vi "commander5.vi"() -> ()   [LabVIEW 2015]
uses:
  G_SEN.vi
  G_NAV.vi
  G_DATA.vi
  G_LCM.vi
  G_VEH.vi
  G_PATH.vi
panel:
  in  "shifthold":dbl=0.0025
  out "String":string="콜 서비스 대기 중"
  out "EURECAR_VISION":T1
  out "count":i32
  out "P2V Sign":picture[](array[picture])=[bytes[7530], bytes[7530], bytes[7530], bytes[7530]]
  out "Array 2":picture[](array[picture])
  out "sign 2":picture[](array[picture])
  out "sign":picture[](array[picture])
  in  "TTL":bool
  in  "Steering gain":dbl=0.8
  in  "half width":dbl=1.9
  out "obs shift":dbl format="%.2f"
  in  "lane keep":bool
  in  "vel":bool
  in  "replay":bool
  in  "x":dbl min=-5.0 max=5.0 step=1.0
  out "lane_shift":dbl=0.06529975046455076
  out "display":u32=10
  out "control":u32=10
  out "update":bool=TRUE
  in  "save lcm":bool
  out "LCM Recv Data":string="GGA_2\t266\rSDT_GPS_DATA\t268\rGGA_1\t268\rRMC_2\t259\rRMC_1\t262\rEYE_RAW_T\t537\rPATH_T\t1344\rIBEO_2202_T\t672\rPOS_T\t3572\rCON_T\t4009\rCAN_T\t4707\r"
  out "GPS DATA 2":T2={"type"="WAAS", "x_lcc"=-395.2637182511565, "y_lcc"=-852.8277788987846, "latdev"=0.99, "londev"=0.99, "sats"=11, "gps_l1_ranges"=0, "gps_l1_mask_ranges"=0, "gps_l2_mask_ranges"=0, "Heading"=151.74409645131422, "lon"=127.35651, "lat"=36.36776, "time"="15:03:34.8", "hgps"=151.54, "lag"=0.0, "MAP"="KAIST"} {"lag" format="%#_5g"; "hgps" format="%#_5g"; "lat" format="%#_11g"; "lon" format="%#_11g"; "Heading" format="%#_5g"; "latdev" format="%#_4g"; "londev" format="%#_4g"}
  in  "Obs":bool=TRUE
  in  "Log":bool
  out "path":u32=10
  out "sensor":u32=10 format="%02.0f"
  out "Speed limit":dbl=20.0
  out "collision":bool
  in  "Load WPT":bool
  in  "Max. Vel.":dbl=20.0 min=-5.0 max=120.0 step=5.0
  in  "RESET PATH":bool
  out "col":i16(graph)
  out "stop":bool
  in  "Reverse":bool
  in  "STOP":bool
  out "Waveform Chart 4":cluster{"auto":i16, "run":i16}(graph)={"auto"=1, "run"=0}
  out "Waveform Chart 3":cluster{"Steer_input":dbl, dbl, "handle":dbl}(graph)
  out "Waveform Chart 2":T3(graph)={"VS_des"=0.0, "VS_can"=31.498562500000002, "VS_des"=20.0}
  out "Heading":cluster{"Heading":dbl, "hgps":dbl}(graph)={"Heading"=151.74409645131422, "hgps"=151.54}
  out "XY Graph 2":cluster{"Y":dbl[], "Y":dbl[]}[](graph)=[{"Y"=[-395.3040396828474], "Y"=[-852.7527551292769]}, {"Y"=array[29298 elements], "Y"=array[29298 elements]}, {"Y"=array[29298 elements], "Y"=array[29298 elements]}, {"Y"=[-390.58210518912017], "Y"=[-861.284610912867]}]
  out "Gauge":cluster{dbl, dbl, dbl}(knob)={0.0, 31.498562500000002, 20.0} scale=-20.0..140.0
  out "Meter":cluster{dbl, dbl, dbl}(knob)={-3.5333877271700453, -5.2, -7.217874503679048} scale=-550.0..550.0
  out "XY Graph":cluster{"Y":dbl[], "Y":dbl[]}[](graph)=[{"Y"=[0.0], "Y"=[0.0]}, {"Y"=array[300 elements], "Y"=array[300 elements]}, {"Y"=[0.0, 0.0, 0.0, 0.0, 0.0, 0.0, 0.0, 0.0, 0.0, 0.0, 0.0, 0.0, 0.0, 0.0, 0.0, 0.0, 0.0, 0.0, 0.0, 0.0, 0.0, 0.0, 0.0, 0.0, 0.0, 0.0, 0.0, 0.0, 0.0, 0.0, 0.0, 0.0, 0.0, 0.0, 0.0, 0.0, 0.0, 0.0, 0.0, 0.0, 0.0, 0.0, 0.0, 0.0, 0.0, 0.0, 0.0, 0.0, 0.0, 0.0, 0.0, 0.0, 0.0, 0.0, 0.0, 0.0, 0.0, 0.0, 0.0, 0.0, 0.0, 0.0, 0.0, 0.0, 0.0, 0.0, 0.0, 0.0, 0.0, 0.0, 0.0, 0.0, 0.0, 0.0, 0.0, 0.0, 0.0, 0.0, 0.0, 0.0, 0.0, 0.0, 0.0, 0.0, 0.0, 0.0, 0.0, 0.0, 0.0, 0.0, 0.0, 0.0, 0.0, 0.0, 0.0, 0.0, 0.0, 0.0, 0.0, 0.0, 0.0, 0.0, 0.0, 0.0, 0.0, 0.0, 0.0, 0.0, 0.0, 0.0, 0.0, 0.0, 0.0, 0.0, 0.0, 0.0, 0.0, 0.0, 0.0, 0.0, 0.0, 0.0, 0.0, 0.0, 0.0, 0.0, 0.0, 0.0, 0.0, 0.0, 0.0, 0.0, 0.0, 0.0, 0.0, 0.0, 0.0, 0.0, 0.0, 0.0, 0.0, 0.0, 0.0, 0.0, 0.0, 0.0, 0.0, 0.0, 0.0, 0.0, 0.0, 0.0, 0.0, 0.0, 0.0, 0.0, 0.0, 0.0, 0.0, 0.0, 0.0, 0.0, 0.0, 0.0, 0.0, 0.0, 0.0, 0.0, 0.0, 0.0, 0.0, 0.0, 0.0, 0.0, 0.0, 0.0, 0.0, 0.0, 0.0, 0.0, 0.0, 0.0, 0.0, 0.0, 0.0, 0.0, 0.0, 0.0, 0.0, 0.0, 0.0, 0.0, 0.0, 0.0, 0.0, 0.0, 0.0, 0.0, 0.0, 0.0, 0.0, 0.0, 0.0, 0.0, 0.0, 0.0, 0.0, 0.0, 0.0, 0.0, 0.0, 0.0, 0.0, 0.0, 0.0, 0.0, 0.0, 0.0, 0.0, 0.0, 0.0, 0.0, 0.0, 0.0, 0.0, 0.0, 0.0, 0.0, 0.0, 0.0, 0.0, 0.0, 0.0, 0.0, 0.0, 0.0, 0.0, 0.0, 0.0, 0.0, 0.0, 0.0, 0.0, 0.0, 0.0, 0.0, 0.0, 0.0, 0.0, 0.0, 0.0, 0.0, 0.0, 0.0, 0.0, 0.0, 0.0, 0.0, 0.0, 0.0, 0.0, 0.0, 0.0, 0.0, 0.0, 0.0, 0.0, 0.0, 0.0, 0.0, 0.0, 0.0, 0.0, 0.0, 0.0, 0.0, 0.0, 0.0, 0.0, 0.0, 0.0, 0.0, 0.0, 0.0, 0.0, 0.0, 0.0, 0.0, 0.0, 0.0, 0.0, 0.0, 0.0, 0.0, 0.0, 0.0, 0.0, 0.0, 0.0, 0.0], "Y"=array[300 elements]}, {"Y"=[2.318130381696859, -0.1745458769952298], "Y"=[11.969202289956298, -0.08456504992216807]}, {"Y"=[-0.010485723266884323], "Y"=[-0.366787169288041]}, {"Y"=[], "Y"=[]}, {"Y"=[0.0, 1.2348716609267285e-05, 4.939486689181649e-05, 0.00011113845039290027, 0.00019757946665777126, 0.00030871791523168213, 0.0004445537956598855, 0.000605087106123392, 0.0007903178461674543, 0.0010002460144278302, 0.0012348716095402779, 0.0014941946296858077, 0.0017782150735001778, 0.0020869329387096514, 0.002420348223495239, 0.0027784609251284564, 0.0031612710417903145, 0.0035687785702975816, 0.004000983508831268, 0.004457885852843901, 0.0049394856009712385, 0.0054457827491205535, 0.005976777293653868, 0.0065324692313879495, 0.00711285855868482, 0.0077179452709970064, 0.00834772936468653, 0.009002210835660662, 0.009681389678462438, 0.010385265889908624, 0.011113839464087505, 0.011867110396906355, 0.012645078682453459, 0.013447744316181343, 0.01427510729217829, 0.015127167604987335, 0.01600392524869676, 0.016905380218304344, 0.017831532506079384, 0.018782382107019657, 0.019757929013849207, 0.02075817322020157, 0.02178311472016503, 0.022832753505554138, 0.023907089570002427, 0.02500612290623394, 0.026129853506063228, 0.02727828136221433, 0.02845140646741129, 0.029649228813468653, 0.030871748391746223, 0.03211896519496804, 0.03339087921358441, 0.03468749043986463, 0.036008798864259006, 0.037354804478127335, 0.03872550727237467, 0.040120907238360815, 0.04154100436517183, 0.042985798644622264, 0.04445529006625293, 0.04594947862005938, 0.04746836429558243, 0.04901194708327239, 0.05058022697267006, 0.052173203952406766, 0.05379087801247806, 0.05543324914151526, 0.057100317328149686, 0.05879208256192214, 0.06050854483009971, 0.06224970412222319, 0.06401556042555967, 0.0658061137291952, 0.06762136402039687, 0.06946131128643174, 0.07132595551547638, 0.07321529669479787, 0.07512933481120854, 0.0770680698524302, 0.07903150180436569, 0.08101963065473683, 0.08303245638944645, 0.08506997899485214, 0.08713219845731146, 0.08921911476272726, 0.09133072789745711, 0.0934670378460396, 0.09562804459574181, 0.09781374813019283, 0.1000241484352955, 0.1022592454964979, 0.10451903929788386, 0.10680352982444674, 0.10911271706117986, 0.11144660099125758, 0.11380518160012798, 0.1161884588709654, 0.11859643278830845, 0.12102910333487671, 0.12348647049520878], "Y"=[0.0, 0.2999999996611315, 0.5999999972890523, 0.8999999908505517, 1.1999999783124187, 1.4999999576414431, 1.799999926804414, 2.0999998837681204, 2.3999998264993527, 2.6999997529649002, 2.9999996611315525, 3.2999995489661003, 3.5999994144353322, 3.8999992555060397, 4.199999070145011, 4.4999988563190385, 4.799998611994914, 5.099998335139425, 5.399998023719366, 5.699997675701526, 5.999997289052697, 6.299996861739673, 6.599996391729244, 6.899995876988203, 7.199995315483342, 7.499994705181453, 7.799994044049336, 8.099993330053774, 8.39999256116157, 8.699991735339516, 8.999990850554404, 9.299989904773033, 9.599988895962198, 9.899987822088692, 10.199986681119317, 10.499985471020864, 10.799984189760135, 11.099982835303924, 11.399981405619032, 11.69997989867226, 11.9999783124304, 12.299976644860262, 12.599974893928637, 12.899973057602335, 13.19997113384815, 13.499969120632889, 13.799967015923354, 14.099964817686345, 14.399962523888673, 14.69996013249714, 14.999957641478545, 15.299955048799703, 15.599952352427417, 15.899949550328495, 16.199946640469744, 16.499943620817973, 16.799940489339992, 17.099937244002618, 17.399933882772654, 17.699930403616914, 17.99992680450221, 18.299923083395356, 18.599919238263176, 18.899915267072465, 19.199911167790056, 19.49990693838276, 19.799902576817402, 20.09989808106079, 20.399893449079745, 20.699888678841095, 20.999883768311655, 21.299878715458252, 21.599873518247712, 21.89986817464685, 22.1998626826225, 22.49985704014148, 22.799851245170622, 23.09984529567676, 23.399839189626718, 23.699832924987327, 23.999826499725415, 24.299819911807823, 24.599813159201382, 24.899806239872923, 25.199799151789286, 25.4997918929173, 25.79978446122382, 26.099776854675675, 26.399769071239707, 26.699761108882754, 26.999752965571663, 27.299744639273282, 27.599736127954454, 27.899727429582022, 28.199718542122838, 28.499709463543752, 28.799700191811617, 29.099690724893275, 29.39968106075559, 29.69967119736542, 29.9996611326896]}, {"Y"=[-0.06600916953808209, -0.06344179564483016, -0.0608518444823114, -0.058239099738796596, -0.05560334510235676, -0.05294436426110516, -0.050261940903320035, -0.047555858717060806, -0.04482590139060627, -0.042071852612023175, -0.039293496069478184, -0.03649061545119325, -0.03366299444539189, -0.030810416740034263, -0.027932666023448238, -0.02502952598375119, -0.022100780309060486, -0.01914621268759653, -0.016165606807529986, -0.013158746356981332, -0.01012541502422426, -0.007065396497267784, -0.003978474464338966, -0.0008644326136044711, 0.0022769453667148554, 0.005445875788548271, 0.008642574963678484, 0.011867259203984126, 0.015120144821300308, 0.018401448127346676, 0.021711385434113772, 0.02505017305337809, 0.028418027296971182, 0.031815164476669544, 0.03524180090440954, 0.038698152891966764, 0.04218443675117278, 0.045700868794012806, 0.049247665332112334, 0.052825042677346445, 0.056433217141655945, 0.060072405036816434], "Y"=[0.5121809097675571, 1.0121752601384235, 1.5121695384012186, 2.012163743865094, 2.512157875839095, 3.0121519336325457, 3.5121459165543456, 4.012139823913919, 4.512133655020165, 5.012127409182253, 5.51212108570941, 6.01211468391076, 6.512108203095302, 7.012101642572408, 7.5120950016510015, 8.012088279640283, 8.512081475849447, 9.012074589587623, 9.512067620163906, 10.012060566887367, 10.512053429067162, 11.01204620601256, 11.512038897032557, 12.012031501436383, 12.512024018533157, 13.012016447631929, 13.512008788041948, 14.012001039072286, 14.511993200032173, 15.011985270230497, 15.511977248976663, 16.01196913557967, 16.51196092934874, 17.011952629592873, 17.511944235621367, 18.01193574674322, 18.511927162267657, 19.01191848150382, 19.511909703760793, 20.011900828347645, 20.511891854573676, 21.01188278174788]}, {"Y"=array[29298 elements], "Y"=array[29298 elements]}, {"Y"=array[300 elements], "Y"=array[300 elements]}, {"Y"=array[300 elements], "Y"=array[300 elements]}, {"Y"=[], "Y"=[]}, {"Y"=[3.0695394261907176, 3.04865065448307, 3.048008216792561, 3.1210527739835254, 3.324526996249824, 2.947243604363593, 2.9701196741924507, 3.2479597439468604, 3.0074095456829615, 3.3404045915050884, 3.312198968398903, 3.3442367518584226, 2.9712191141581634, 3.312230782027615, 3.2131015151472186, 2.9523788068661134, 3.2454016157352643, 3.35871965215567, 3.2429958584944476, 3.219399826058981, 3.208921836311342, 3.234549978178593, 3.285982291082405, 3.20449286569777, 3.3973553285568197, 3.4101498412097295, 3.3776012113068528, 3.552175301464521, 3.4914449694264804, 3.443582315332557, 3.550578979032941, 3.40785022669485, 3.436692573868031, 3.741413780021891, 3.475131019765175, 3.743662660021443, 3.6000120434228204, 2.468319752067167, 2.625655513798486, 2.4548984007767616, 2.617756495329653, 2.580363244114453, 2.4673140153981747, 2.5674673044097025, 2.4632390127360324, 2.551735063331595, 2.467662926036525, 2.545504745981361, -6.014099257028617, -5.98866059593555, 2.5327580439291943, -5.976017599211303, 2.467908566874166, -5.893118654752842, -5.850615620997258, -5.66266820570784, -5.78971714096454, -5.853735779721767, 2.516656099985925, 2.4412912316361193, -5.6612111316482965, 2.945308269064661, 2.318130381696859, -5.816199239066796, -5.645557045890771, -5.789161989467775, 2.494355053763526, -5.640953706533398, 2.444819798705696, -5.811841135661254, -5.756911264222725, -5.646985418361251, 2.9646433902149365, 2.902044742092418, -5.76980024321233, -5.71912936315645, -5.663231049359712, -5.641219287611779, -5.740709863823967, -5.6296797206314455, 2.901151351508035, -5.723858315344926, -5.687639186304427, -5.651648796973401, 2.8716850870712514, -5.636308173138567, -5.708993389959358, -5.6756050416330925, -5.630713620049172, -5.686764195715769, 2.874899644034143, -5.672867876096028, -5.685030680901294, -5.6615229389822295, -5.6689161799689485, -5.66295649358774, 3.3435270664923835, -5.681120270583116, 3.4189618675175746, 2.61741991105427, 2.4954314772037374, -5.667713825528187, -5.620189164651901, -5.642823168306656, -5.668824101802754, -5.6121502897582, -5.607168890864395, 2.6354904855004824, -8.237185254375097, -8.393839405035447, 2.502361285636947, -8.13992618825447, -5.5538278385477735, -5.5832462000900245, -5.551545962942625, -5.588011576946744, -5.565804135535585, -5.602371953404233, -5.593738753494274, -5.628995192627058, -5.614561921601172, -5.6222785656109115, -5.634079222000596, -5.570781709227749, -5.622494988286693, -5.5726939302833225, 2.547952790334438], "Y"=[6.604466382759696, 6.638746684564207, 6.6946194868131155, 6.656886746310402, 6.576797332581769, 6.970487136791295, 6.966105810136174, 6.727959743946861, 6.9471473492896205, 6.647373824165766, 6.676837802450745, 6.679274813811849, 7.030548733312288, 6.734054987461864, 6.8386803125046285, 7.072176735761396, 6.842488269208289, 6.750627670193209, 6.900093588313969, 6.936002074025792, 6.986489104286848, 6.983206148071301, 6.976253615707609, 7.044480506066268, 6.9075712124628765, 6.981943166952128, 7.010518936926658, 6.878332670246209, 6.9406740998976595, 7.0162625616212795, 6.937528751721111, 7.105803046608284, 7.201882776091162, 7.1884709841399825, 7.449641539449491, 7.256913909048313, 7.448349880172145, 10.541515597925486, 10.58636574754925, 10.704753183008643, 10.75960073152162, 10.857916658865527, 10.953458544322455, 11.031677017427471, 11.164954334484273, 11.205766460820067, 11.415006650319999, 11.41814222736707, 9.49911149637188, 9.579663070404832, 11.621461987887608, 9.674719568114075, 11.665707829064013, 9.80664506068822, 9.872236302393265, 10.118917498191617, 10.032789265350505, 9.989929971746363, 11.825153825387254, 11.8404582472012, 10.236943413135462, 11.772624531275717, 11.969202289956298, 10.18135187717981, 10.339937485200185, 10.269666919428355, 12.01959870848977, 10.458792124392044, 12.130470600786513, 10.419672219730087, 10.477448492786499, 10.593814651738162, 12.062612923648652, 12.126443379373132, 10.620774421116442, 10.686154690192177, 10.745305127145643, 10.84979860216937, 10.846277484013116, 10.970504371012535, 12.379648081257772, 10.959464295986388, 11.048832093414353, 11.140008128983286, 12.55734161946395, 11.26171521575083, 11.218936190005936, 11.31680739351499, 11.400085032671795, 11.480133550586793, 12.849716260084092, 11.611323526751976, 11.784276543876027, 11.908086345991677, 12.08237216014506, 12.240576852972636, 13.427008368241497, 12.441676206197144, 13.949957882106105, 14.330845448197648, 14.455475033151467, 14.821596735952657, 14.978197356946716, 15.28848192570302, 15.61817167132016, 16.376255434010254, 16.68234363463669, 21.95150547106146, 20.40379179066285, 20.349632555825004, 22.184396062486776, 20.58309792509196, 22.945101475785034, 23.04941111765418, 23.609436944190787, 23.743191267681656, 24.38049164670381, 11.661729940781953, 11.966609075046962, 12.358258644115107, 14.839042684564758, 15.112524959067793, 15.405096536253911, 15.54424982037931, 16.557975501696212, 16.762962587325568, 23.85157748746847]}, {"Y"=array[4151 elements], "Y"=array[4151 elements]}, {"Y"=[3.3176839012103994, 3.2928246247771895, 3.217016245471217, 3.1370987639973738, 3.075304658021821, 2.6343108252190195, 2.6178268757305325, 2.599590896624237, 2.5961493744296433, -5.493730202945327, -5.499603600475432, -5.503348882486225, -5.518288804571267, -5.528340978901209, -5.5360266600129595, -5.543967730902173, -5.548647916044711, -5.550062138140339, -5.555504675699071, -5.55911775283573, -5.565164072400016, -5.572005900149632, -7.82045425071548, -7.9036920393673835, -8.25752605699809], "Y"=[29.22041127625098, 23.27485457149493, 23.975155866595713, 29.675700343851595, 25.712976152685094, 35.05095860577215, 31.780818790794022, 29.060764892809168, 26.909910954479866, 40.298306961951944, 34.46758759193476, 38.18422498046205, 36.32954522138188, 31.607667334900388, 33.090708024367146, 30.372314208018064, 29.18791605000413, 28.083784709400362, 25.250907275648988, 27.098733562358454, 26.17391273348185, 24.494648004120613, 26.316192633652083, 25.88774384104577, 24.998902406387412]}, {"Y"=[-0.925, -0.925, -0.925, -0.6775, -0.6775, -0.925, -0.925, -0.925, -0.925, -0.6775, -0.6775, -0.925, -0.925, -0.925, 0.9025, 0.9025, 0.9025, 0.6775, 0.6775, 0.9025, 0.9025, 0.9025, 0.9025, 0.6775, 0.6775, 0.9025, 0.9025, 0.9025, -0.925], "Y"=[-0.75, -0.224, 0.224, 0.224, -0.224, -0.224, 0.224, 2.415, 2.885, 2.885, 2.415, 2.415, 2.885, 3.5, 3.5, 2.885, 2.415, 2.415, 2.885, 2.885, 2.415, 0.224, -0.224, -0.224, 0.224, 0.224, -0.224, -0.75, -0.75]}, {"Y"=[-1.989725401977954], "Y"=[16.427453516317758]}]
  in  "Make WPT":bool
  # "V2I Traffic Signal"
  # "CNN\nSign\nDetection"
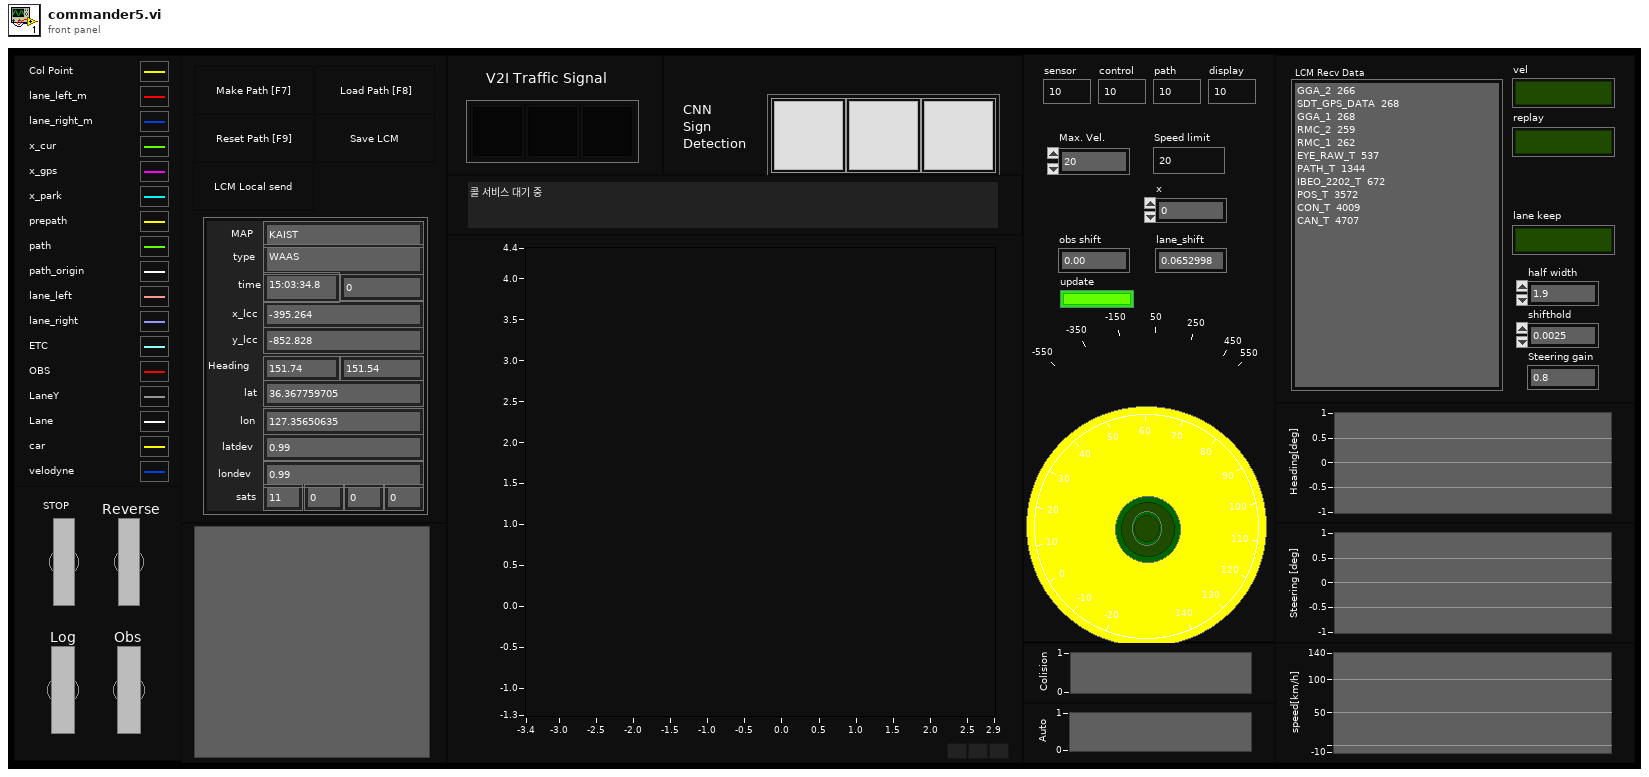
[diagram p1: front panel]
types:
  T1 = cluster{"hash":i64, "sys time":i64, "status":i32, "TS_num":i32, "TS_type":i32[], "TS_loc_x":dbl[], "TS_loc_y":dbl[]}
  T2 = cluster{"type":string, "x_lcc":dbl, "y_lcc":dbl, "latdev":sgl, "londev":sgl, "sats":u8, "gps_l1_ranges":u8, "gps_l1_mask_ranges":u8, "gps_l2_mask_ranges":u8, "Heading":dbl, "lon":sgl, "lat":sgl, "time":string, "hgps":dbl, "lag":dbl, "MAP":string}
  T3 = cluster{"VS_des":dbl, "VS_can":dbl, "VS_des":dbl}
  T4 = enum8{"Enabled", "Disabled", "Disabled and Grayed Out"}
  T5 = cluster{"idx":i32, "x":dbl, "y":dbl, "h":dbl, "x_path":dbl}
  T6 = cluster{"idx":i32, "x":dbl, "y":dbl, "hp":dbl, "x_path":dbl}
  T7 = cluster{"X":cluster{"idx":i32, "x":dbl, "y":dbl, "h":dbl, "x_path":dbl}}[]
  T8 = typedef "imagedata.ctl" = cluster{"image type":i32, "image depth":i32, "image":u8[], "mask":u8[], "colors":u32[], "Rectangle":cluster{"left":i16, "top":i16, "right":i16, "bottom":i16}}
  T9 = cluster{"hash":i64, "sys time":i64, "s_lat":dbl, "s_lon":dbl, "d_lat":dbl, "d_lon":dbl, "Message":i64}
  T10 = cluster{"Steer_input":dbl, "Steer_output":dbl, "VS_des":dbl, "VS_can":dbl, "heading":dbl, "auto":bool, "run":bool, "x":dbl, "y":dbl}
  T11 = cluster{"GPSTime":dbl, "attitude[2]":dbl, "lcc[0]":dbl, "lcc[1]":dbl, "heading_GPS":dbl}
  T12 = cluster{"Minimum":dbl, "Minimum":dbl, "Minimum":dbl, "Minimum":dbl, "Minimum":dbl}
  T13 = cluster{"X":cluster{"c_idx":i32, "xc":dbl, "yc":dbl, "hc":dbl, "xc_path":dbl}}[]
  T14 = cluster{"hash":i64, "sys time":i64, "time":dbl, "x":dbl, "y":dbl, "h":dbl, "numSV":i32, "postype":i32, "lag":i32, "hordev":dbl, "lat":dbl, "lon":dbl, "hgt":dbl, "map_idx":i32}
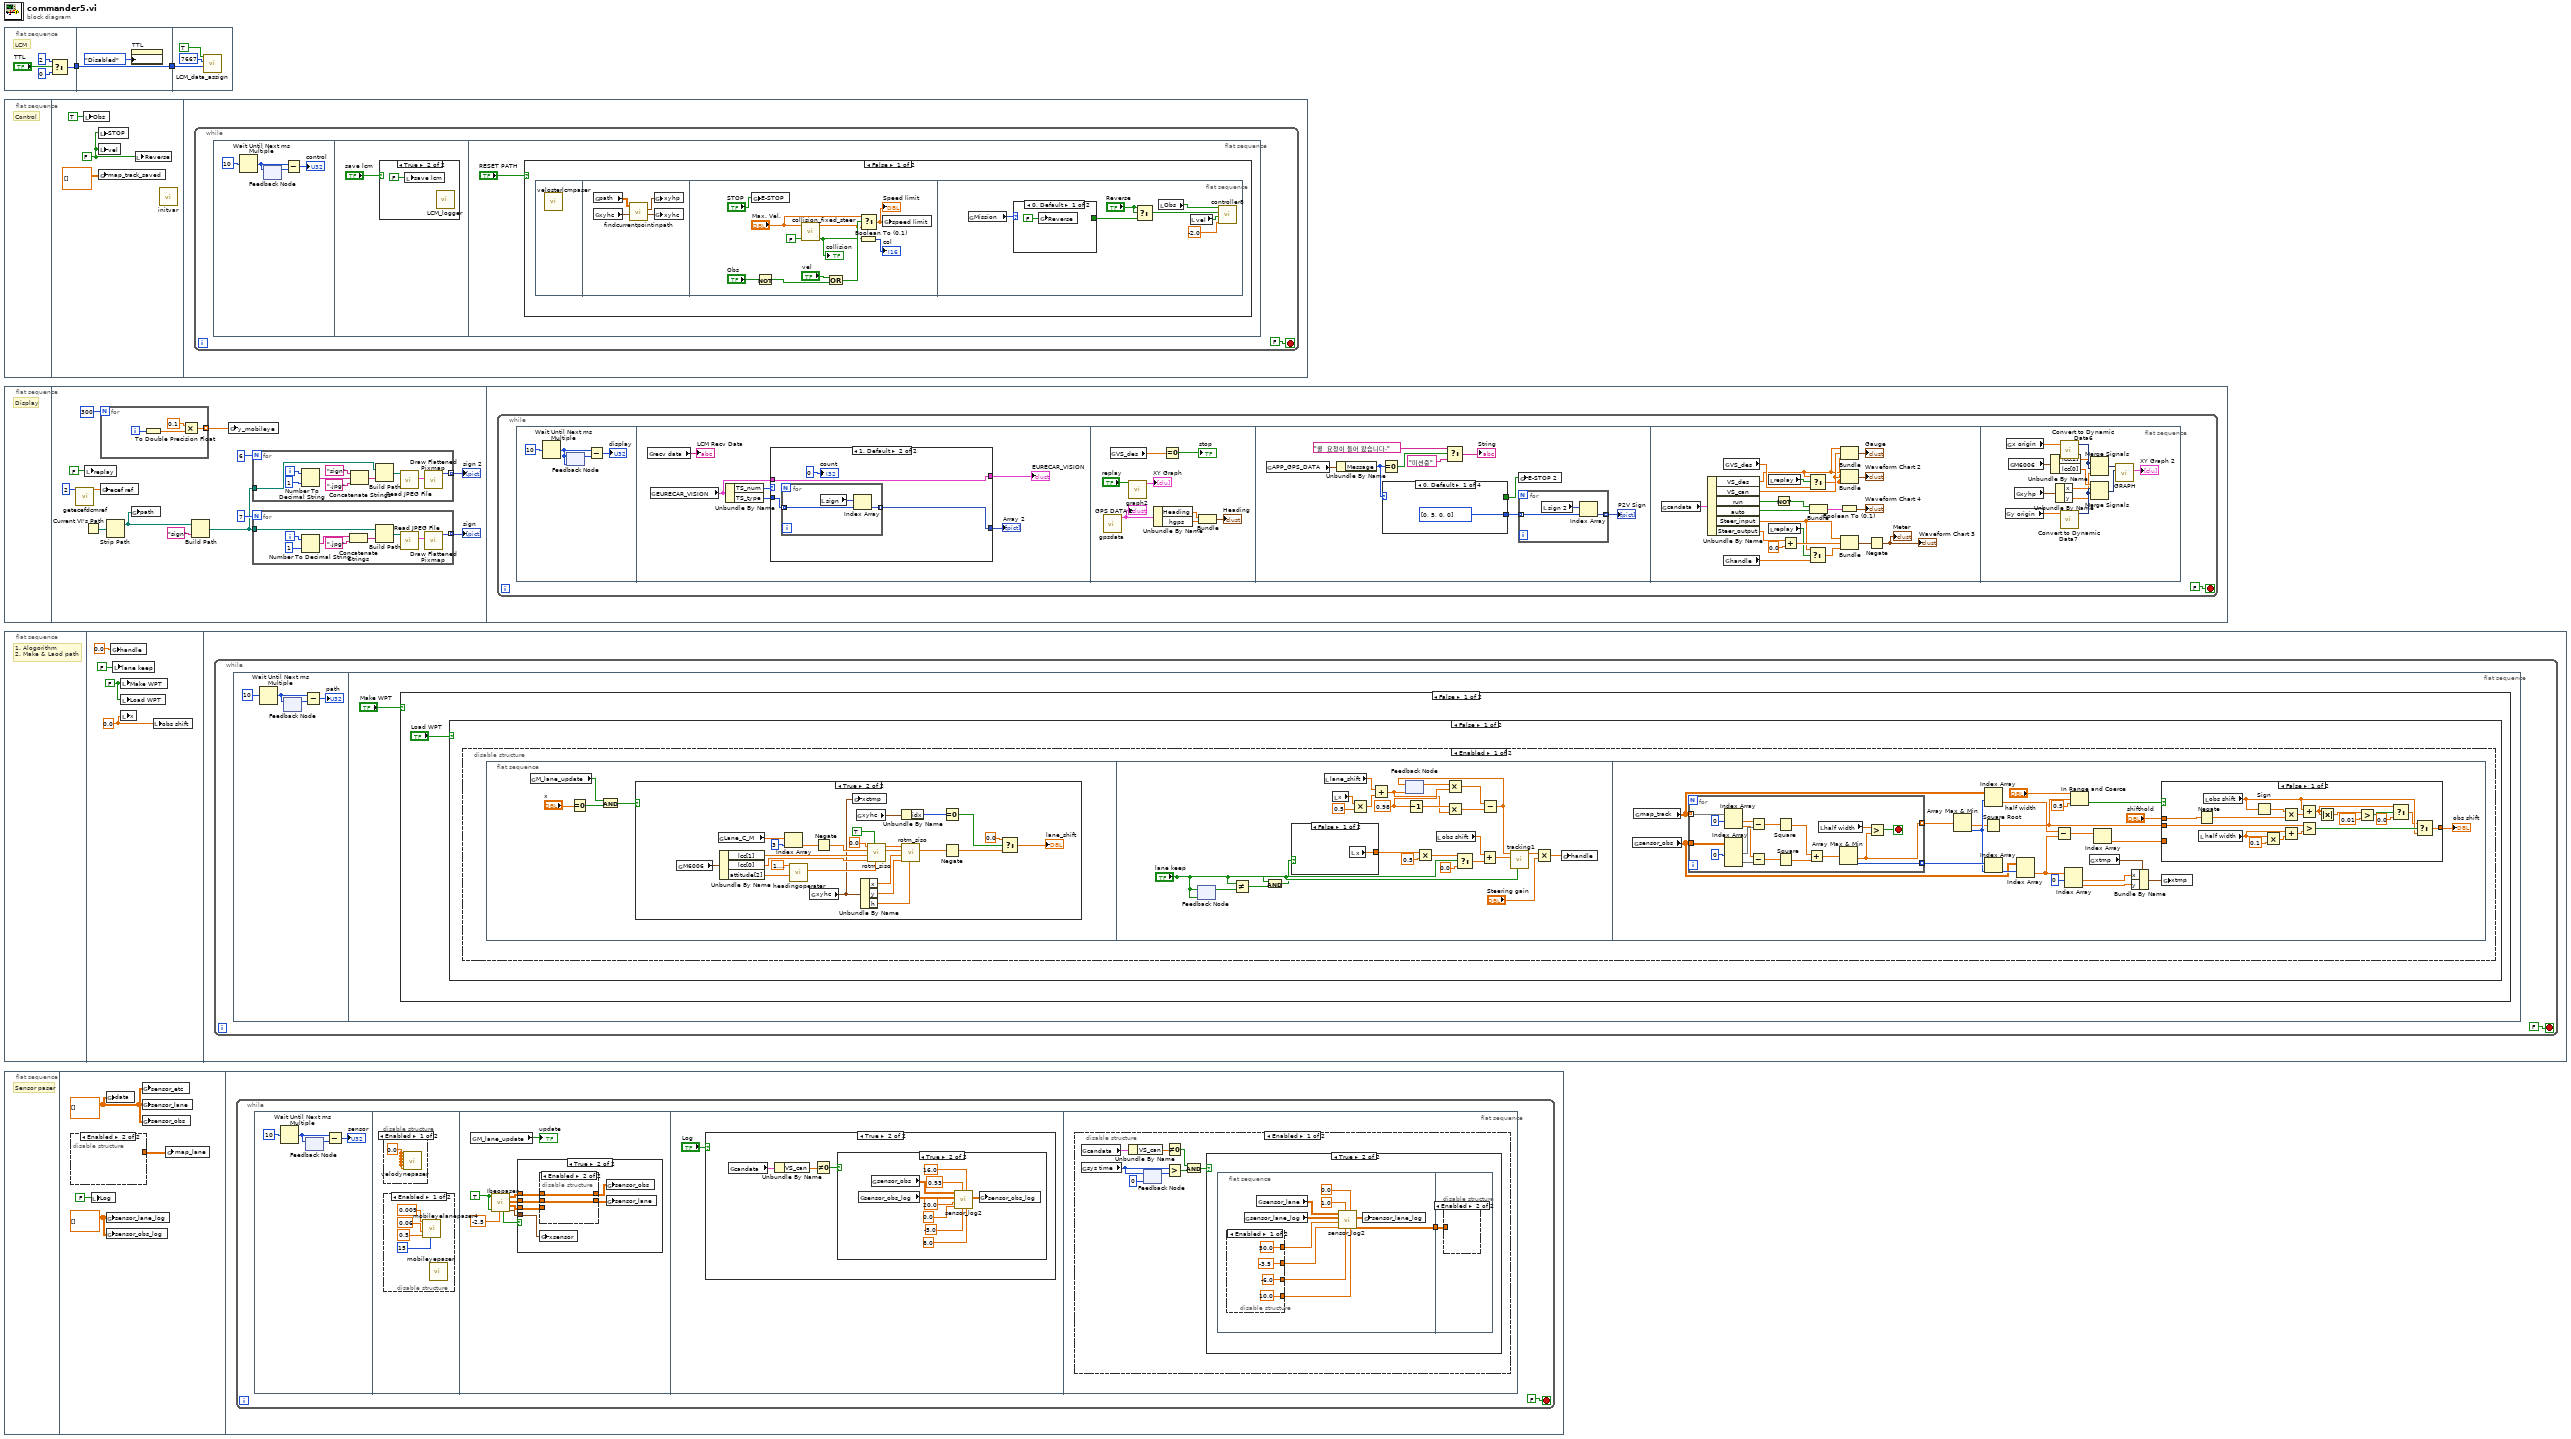
[diagram p0: block diagram]
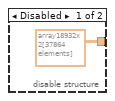
[diagram p2: hidden frame]
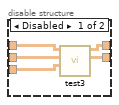
[diagram p6: hidden frame]
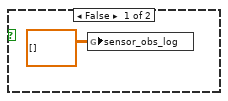
[diagram p7: hidden frame]
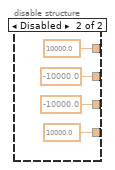
[diagram p10: hidden frame]
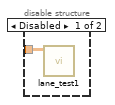
[diagram p11: hidden frame]
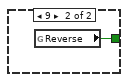
[diagram p14: hidden frame]
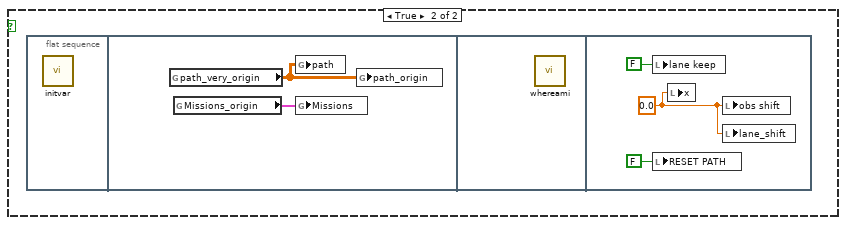
[diagram p15: hidden frame]
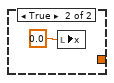
[diagram p17: hidden frame]
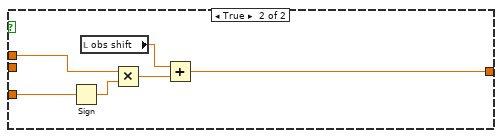
[diagram p18: hidden frame]
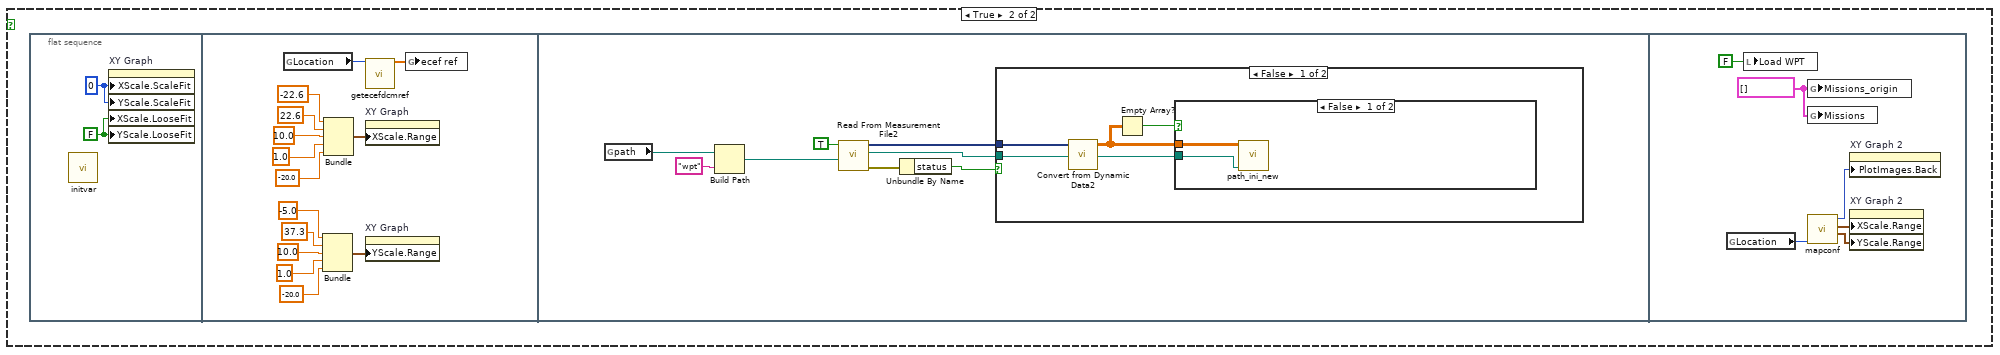
[diagram p20: hidden frame]
diagram:
  n1 = flat-sequence {
    tunnel: [w3] -> w1
    tunnel: [w8] -> w2
    tunnel: w1 -> [w8]
    tunnel: w2 -> [w11]
    frame #0 {
      # "LCM"
      n2 = Select(t=u16 2 ("time-to-live"), s="TTL", f=u16 0 ("time-to-live")) -> (s? t:f=w3:u16)
    }
    frame #1 {
      n3 = property on="TTL" class="Bool (strict)"("DisabledEnum"=T4."Disabled" ("Disabled")) -> ()  [unwired: 2 in, 2 out]
    }
    frame #2 {
      n4 = call "LCM_data_assign.vi"("time-to-live"=w11, "port"=u16 7667, "velodyne enable"=TRUE) -> ()  [unwired: 9 in]
    }
  }
  n5 = flat-sequence {
    frame #0 {
      # "Control"
    }
    frame #1 {
      w13 = FALSE ("LCM")
      n6 = local write "Obs"(TRUE ("obs")) -> ()
      n7 = local write "STOP"(w13) -> ()
      n8 = local write "vel"(w13) -> ()
      n9 = global write "G_PATH.vi" "map_track_saved"(dbl[][] [] ("map_track_saved")) -> ()
      n10 = local write "Reverse"(w13) -> ()
      n11 = call "initvar.vi"() -> ()  [unwired: 12 in]
    }
    frame #2 {
      n12 = while {
        stop <- FALSE ("Boolean") stop-if-true
        n13 = flat-sequence {
          frame #0 {
            n14 = Wait Until Next ms Multiple(millisecond multiple=u32 10 ("milliseconds to wait")) -> (millisecond timer value=w16:u32)
            n15 = feedback #1() -> (w17:u32)  [unwired: 1 in]
            n16 = feedback-in #1(w16) -> ()
            n17 = Subtract(x=w16, y=w17) -> (x-y=→"control":u32)
          }
          frame #1 {
            n18 = case shown="True" "save lcm" {
              frame False {
              }
              frame True {
                n19 = local write "save lcm"(FALSE ("save lcm")) -> ()
                n20 = call "LCM_logger.vi"() -> ()  [unwired: 12 in]
              }
            }
          }
          frame #2 {
            n21 = case shown="False" "RESET PATH" {
              frame False {
                n22 = flat-sequence {
                  frame #0 {
                    n23 = call "velosterlcmpaser.vi"() -> ()  [unwired: 11 in, 1 out]
                  }
                  frame #1 {
                    n24 = global read "G_PATH.vi" "path"() -> (w24:dbl[][])
                    n25 = global read "G_VEH.vi" "xyhc"() -> (w25:T5)
                    n26 = call "findcurrentpointinpath.vi"("xyhc_in"=w25, "path_updated"=w24) -> ("xyhc_out"=w23:T5, "xyhp"=w26:T6)  [unwired: 8 in]
                    n27 = global write "G_VEH.vi" "xyhp"(w26) -> ()
                    n28 = global write "G_VEH.vi" "xyhc"(w23) -> ()
                  }
                  frame #2 {
                    n29 = global write "G_VEH.vi" "E-STOP"("STOP") -> ()
                    n30 = Not(x="Obs") -> (.not. x?=w35:bool)
                    n31 = call "collision_fixed_steer.vi"("obsclose"=FALSE, "Max. Vel."="Max. Vel.") -> ("collision"=w27:bool, "speed limit"=w32:dbl)  [unwired: 8 in]
                    "collision" <- w27
                    n32 = Or(x="vel", y=w35) -> (x .or. y?=w37:bool)
                    n33 = Boolean To (0,1)(Boolean=w27) -> (0, 1=→"col":i16)
                    n34 = Select(t="Max. Vel.", s=w37, f=w32) -> (s? t:f=w33:dbl)
                    "Speed limit" <- w33
                    n35 = global write "G_VEH.vi" "speed limit"(w33) -> ()
                  }
                  frame #3 {
                    n36 = global read "G_PATH.vi" "Mission"() -> (w42:i32)
                    n37 = case shown="0, Default" w42 {
                      tunnel: [_ w46] -> w39
                      frame 0, Default {
                        n38 = global write "G_VEH.vi" "Reverse"(FALSE ("Reverse")) -> ()
                      }
                      frame 9 {
                        n39 = global read "G_VEH.vi" "Reverse"() -> (w46:bool)
                      }
                    }
                    n40 = Select(t="Reverse", s="Reverse", f=w39) -> (s? t:f=w40:bool)
                    n41 = local read "Obs"() -> (w43:bool)
                    n42 = local read "vel"() -> (w44:bool)
                    n43 = call "controller8.vi"("Neg max speed"=-2.0, "vel"=w44, "reverse"=w40, "obs"=w43) -> ()  [unwired: 8 in]
                  }
                }
              }
              frame True {
                n44 = flat-sequence {
                  frame #0 {
                    n45 = call "initvar.vi"() -> ()  [unwired: 12 in]
                  }
                  frame #1 {
                    n46 = global read "G_PATH.vi" "path_very_origin"() -> (w48:dbl[][])
                    n47 = global read "G_PATH.vi" "Missions_origin"() -> (w47:T7)
                    n48 = global write "G_PATH.vi" "path"(w48) -> ()
                    n49 = global write "G_PATH.vi" "Missions"(w47) -> ()
                    n50 = global write "G_PATH.vi" "path_origin"(w48) -> ()
                  }
                  frame #2 {
                    n51 = call "whereami.vi"() -> ()  [unwired: 12 in]
                  }
                  frame #3 {
                    w49 = 0.0 ("x")
                    n52 = local write "lane keep"(FALSE ("lane keep")) -> ()
                    n53 = local write "RESET PATH"(FALSE ("RESET PATH")) -> ()
                    n54 = local write "x"(w49) -> ()
                    n55 = local write "obs shift"(w49) -> ()
                    n56 = local write "lane_shift"(w49) -> ()
                  }
                }
              }
            }
          }
        }
      }
    }
  }
  n57 = flat-sequence {
    frame #0 {
      # "Display"
    }
    frame #1 {
      n58 = call "getecefdcmref.vi"("map"=2) -> ("XYZ"=w54:dbl[])  [unwired: 10 in, 4 out]
      n59 = local write "replay"(FALSE ("replay")) -> ()
      n60 = Current VI's Path() -> (path=w61:path)
      n61 = for {
        N: 300 -> [_]
        tunnel: [w84] -> w64 mode=indexing
        i -> [w87]
        n62 = To Double Precision Float(number=w87) -> (double precision float=w86:dbl)
        n63 = Multiply(x=0.1, y=w86) -> (x*y=w84:dbl)
      }
      n64 = global write "G_NAV.vi" "ecef ref"(w54) -> ()
      n65 = Strip Path(path=w61) -> (stripped path=w52:path)  [unwired: 1 out]
      n66 = global write "G_DATA.vi" "path"(w52) -> ()
      n67 = Build Path(base path=w52, name or relative path="sign") -> (appended path=w55:path)
      n68 = global write "G_SEN.vi" "y_mobileye"(w64) -> ()
      n69 = for {
        N: 6 -> [_]
        tunnel: [w73] -> w57 mode=indexing
        tunnel: w55 -> [w68]
        i -> [w72]
        n70 = Number To Decimal String(number=w72, width (-)=i16 1) -> (decimal integer string=w70:string)
        n71 = Concatenate Strings("sign" ("string"), w70, ".jpg") -> (w67:string)
        n72 = Build Path(base path=w68, name or relative path=w67) -> (appended path=w66:path)
        n73 = call <vilib>:"Read JPEG File.vi"("path to JPEG file"=w66) -> ("image data"=w74:T8)  [unwired: 8 in, 2 out]
        n74 = call <vilib>:"Draw Flattened Pixmap.vi"("image data"=w74) -> ("new picture"=w73:picture)  [unwired: 8 in]
      }
      "sign 2" <- w57
      n75 = for {
        N: 7 -> [_]
        tunnel: [w82] -> w58 mode=indexing
        tunnel: w55 -> [w77]
        i -> [w81]
        n76 = Number To Decimal String(number=w81, width (-)=i16 1) -> (decimal integer string=w79:string)
        n77 = Concatenate Strings(w79, ".jpg") -> (w76:string)
        n78 = Build Path(base path=w77, name or relative path=w76) -> (appended path=w75:path)
        n79 = call <vilib>:"Read JPEG File.vi"("path to JPEG file"=w75) -> ("image data"=w83:T8)  [unwired: 8 in, 2 out]
        n80 = call <vilib>:"Draw Flattened Pixmap.vi"("image data"=w83) -> ("new picture"=w82:picture)  [unwired: 8 in]
      }
      "sign" <- w58
    }
    frame #2 {
      n81 = while {
        stop <- FALSE ("exit") stop-if-true
        n82 = flat-sequence {
          frame #0 {
            n83 = Wait Until Next ms Multiple(millisecond multiple=u32 10 ("milliseconds to wait")) -> (millisecond timer value=w89:u32)
            n84 = feedback #2(w89) -> (w91:u32)
            n85 = feedback-in #2(w89) -> ()
            n86 = Subtract(x=w89, y=w91) -> (x-y=→"display":u32)
          }
          frame #1 {
            n87 = global read "G_LCM.vi" "recv data"() -> (→"LCM Recv Data":string)
            n88 = global read "G_LCM.vi" "EURECAR_VISION"() -> (w94:T1)
            n89 = Unbundle By Name(w94) -> ("TS_num"=w97:i32, "TS_type"=w96:i32[])
            n90 = case shown="1, Default" w97 {
              tunnel: w96 -> [_ w113]
              tunnel: [w106 w112] -> w95
              tunnel: w94 -> [_ w110]
              tunnel: [w99 w110] -> w93
              frame 0 {
                w108 = 100 ("x")
                n91 = local read "count"() -> (w109:i32)
                n92 = Increment(x=w109) -> (x+1=w104:i32)
                n93 = Max & Min(x=w108, y=w104) -> (min(x,y)=w103:i32)  [unwired: 1 out]
                n94 = local read "EURECAR_VISION"() -> (w100:T1)
                n95 = local write "count"(w103) -> ()
                n96 = Equal?(x=w108, y=w103) -> (x = y?=w102:bool)
                n97 = local read "Array 2"() -> (w105:picture[])
                n98 = Select(t=T1 {"hash"=0, "sys time"=0, "status"=0, "TS_num"=0, "TS_type"=[], "TS_loc_x"=[], "TS_loc_y"=[]} ("EURECAR_VISION"), s=w102, f=w100) -> (s? t:f=w99:T1)
                n99 = Select(t=picture[] [], s=w102, f=w105) -> (s? t:f=w106:picture[])
              }
              frame 1, Default {
                n100 = for {
                  tunnel: w113 -> [w115] mode=indexing
                  tunnel: [w114] -> w112 mode=indexing
                  n101 = local read "sign"() -> (w116:picture[])
                  n102 = Index Array(array=w116, index=w115) -> (element=w114:picture)
                }
                "count" <- 0 ("Numeric Control")
              }
            }
            "Array 2" <- w95
            "EURECAR_VISION" <- w93
          }
          frame #2 {
            n103 = call "gpsdata.vi"() -> ("GPS DATA 2"=w122:T2)  [unwired: 11 in]
            "GPS DATA 2" <- w122
            n104 = global read "G_VEH.vi" "VS_des"() -> (w118:dbl)
            n105 = call "graph2.vi"("replay"="replay") -> ("XY Graph"=→"XY Graph":cluster{"Y":dbl[], "Y":dbl[]}[])  [unwired: 9 in, 1 out]
            n106 = Unbundle By Name(w122) -> ("Heading"=w124:dbl, "hgps"=w123:dbl)
            n107 = Equal To 0?(x=w118) -> (x = 0?=→"stop":bool)
            n108 = Bundle("Heading"=w124, "hgps"=w123) -> (→"Heading":cluster{"Heading":dbl, "hgps":dbl})  [unwired: 1 in]
          }
          frame #3 {
            n109 = global read "G_LCM.vi" "APP_GPS_DATA"() -> (w130:T9)
            n110 = Unbundle By Name(w130) -> ("Message"=w129:i64)
            n111 = Equal To 0?(x=w129) -> (x = 0?=w128:bool)
            n112 = case shown="0, Default" w129 {
              tunnel: [_ TRUE _ _] -> w133
              tunnel: [i32[] [0, 5, 0, 0] i32[] [1, 5, 0, 0] i32[] [0, 2, 0, 0] i32[] [0, 5, 3, 0]] -> w132
              frame 0, Default {
              }
              frame 1 {
              }
              frame 2 {
              }
              frame 3 {
              }
            }
            n113 = Select(t="콜  요청이 들어 왔습니다.", s=w128, f="미션중") -> (s? t:f=→"String":string)
            n114 = global write "G_VEH.vi" "E-STOP 2"(w133) -> ()
            n115 = for {
              tunnel: w132 -> [w140] mode=indexing
              tunnel: [w139] -> w131 mode=indexing
              n116 = local read "sign 2"() -> (w141:picture[])
              n117 = Index Array(array=w141, index=w140) -> (element=w139:picture)
            }
            "P2V Sign" <- w131
          }
          frame #4 {
            n118 = global read "G_VEH.vi" "candata"() -> (w163:T10)
            n119 = Unbundle By Name(w163) -> ("VS_des"=w144:dbl, "VS_can"=w156:dbl, "run"=w154:bool, "auto"=w155:bool, "Steer_input"=w148:dbl, "Steer_output"=w153:dbl)
            n120 = global read "G_VEH.vi" "VS_des"() -> (w145:dbl)
            n121 = global read "G_VEH.vi" "handle"() -> (w149:dbl)
            n122 = local read "replay"() -> (w146:bool)
            n123 = local read "replay"() -> (w150:bool)
            n124 = Not(x=w154) -> (.not. x?=w158:bool)
            n125 = Add(x=w153, y=0.0) -> (x+y=w151:dbl)
            n126 = Select(t=w148, s=w150, f=w149) -> (s? t:f=w147:dbl)
            n127 = Select(t=w144, s=w146, f=w145) -> (s? t:f=w143:dbl)
            n128 = Bundle(w158, "auto"=w155) -> (w160:cluster{bool, "auto":bool})  [unwired: 1 in]
            n129 = Boolean To (0,1)(Boolean=w160) -> (0, 1=→"Waveform Chart 4":cluster{i16, "auto":i16})
            n130 = Bundle("VS_des"=w144, "VS_can"=w156, "VS_des"=w143) -> (→"Gauge":T3)  [unwired: 1 in]
            n131 = Bundle("VS_des"=w144, "VS_can"=w156, "VS_des"=w143) -> (→"Waveform Chart 2":T3)  [unwired: 1 in]
            n132 = Bundle("Steer_input"=w148, w151, "handle"=w147) -> (w162:cluster{"Steer_input":dbl, dbl, "handle":dbl})  [unwired: 1 in]
            n133 = Negate(x=w162) -> (-x=→"Meter" →"Waveform Chart 3":cluster{"Steer_input":dbl, dbl, "handle":dbl})
          }
          frame #5 {
            n134 = global read "G_PATH.vi" "y origin"() -> (w167:dbl[])
            n135 = global read "G_PATH.vi" "x origin"() -> (w168:dbl[])
            n136 = global read "G_NAV.vi" "M6006"() -> (w172:T11)
            n137 = global read "G_VEH.vi" "xyhp"() -> (w166:T5)
            n138 = Unbundle By Name(w172) -> ("lcc[1]"=w173:dbl, "lcc[0]"=w174:dbl)
            n139 = Unbundle By Name(w166) -> ("x"=w170:dbl, "y"=w169:dbl)
            n140 = call "Convert to Dynamic Data6"("Array"=w168) -> ("Dynamic Data Type"=w176:dynamicdata)  [unwired: 3 in]
            n141 = call "Convert to Dynamic Data7"("Array"=w167) -> ("Dynamic Data Type"=w175:dynamicdata)  [unwired: 3 in]
            n142 = Merge Signals(w173, w176, w176, w170) -> (w165:dynamicdata)
            n143 = Merge Signals(w174, w175, w175, w169) -> (w164:dynamicdata)
            n144 = call "GRAPH"("Y Input"=w164, "X Input"=w165) -> ("XY Graph"=→"XY Graph 2":cluster{"Y":dbl[], "Y":dbl[]}[])  [unwired: 3 in, 6 out]
          }
        }
      }
    }
  }
  n145 = flat-sequence {
    frame #0 {
      # "1. Alogorithm\n2. Make & Laod path"
    }
    frame #1 {
      w177 = 0.0 ("x")
      w180 = FALSE ("Make WPT")
      n146 = global write "G_VEH.vi" "handle"(0.0 ("handle")) -> ()
      n147 = local write "lane keep"(FALSE ("lane update")) -> ()
      n148 = local write "Make WPT"(w180) -> ()
      n149 = local write "Load WPT"(w180) -> ()
      n150 = local write "x"(w177) -> ()
      n151 = local write "obs shift"(w177) -> ()
    }
    frame #2 {
      n152 = while {
        stop <- FALSE stop-if-true
        n153 = flat-sequence {
          frame #0 {
            n154 = Wait Until Next ms Multiple(millisecond multiple=u32 10 ("milliseconds to wait")) -> (millisecond timer value=w182:u32)
            n155 = feedback #3() -> (w184:u32)  [unwired: 1 in]
            n156 = feedback-in #3(w182) -> ()
            n157 = Subtract(x=w182, y=w184) -> (x-y=→"path":u32)
          }
          frame #1 {
            n158 = case shown="False" "Make WPT" {
              frame False {
                n159 = case shown="False" "Load WPT" {
                  frame False {
                    n160 = disable-structure shown="Enabled" {
                      frame Enabled {
                        n161 = flat-sequence {
                          frame #0 {
                            n162 = global read "G_SEN.vi" "M_lane_update"() -> (w190:bool)
                            n163 = Equal To 0?(x="x") -> (x = 0?=w189:bool)
                            n164 = And(x=w190, y=w189) -> (x .and. y?=w191:bool)
                            n165 = case shown="True" w191 {
                              frame False {
                              }
                              frame True {
                                n166 = global read "G_NAV.vi" "M6006"() -> (w213:T11)
                                n167 = global read "G_SEN.vi" "Lane_C_M"() -> (w216:dbl[])
                                n168 = Unbundle By Name(w213) -> ("lcc[1]"=w212:dbl, "lcc[0]"=w211:dbl, "attitude[2]"=w209:dbl)
                                n169 = Index Array(array=w216, index=3) -> (element=w202:dbl)
                                n170 = call "headingoperater.vi"("h1"=w209, "h2"=1.5707963267948966) -> ("h2-h1"=w208:dbl)  [unwired: 8 in, 1 out]
                                n171 = global read "G_VEH.vi" "xyhc"() -> (w192:T5)
                                n172 = Negate(x=w202) -> (-x=w207:dbl)
                                n173 = global write "G_VEH.vi" "xctmp"(w192) -> ()
                                n174 = global read "G_VEH.vi" "xyhc"() -> (w214:T5)
                                n175 = Unbundle By Name(w192) -> ("x"=w201:dbl, "y"=w200:dbl, "h"=w199:dbl)
                                n176 = call "rotm_siso.vi"("angle[rad]"=w208, "reverse"=TRUE, "y0"=w211, "x0"=w212, "y"=w207, "x"=0.0) -> ("y'"=w203:dbl, "x'"=w204:dbl)  [unwired: 4 in]
                                n177 = Unbundle By Name(w214) -> ("idx"=w197:i32)
                                n178 = call "rotm_siso.vi"("angle[rad]"=w199, "y0"=w200, "x0"=w201, "y"=w203, "x"=w204) -> ("y'"=w198:dbl)  [unwired: 5 in, 1 out]
                                n179 = Equal To 0?(x=w197) -> (x = 0?=w196:bool)
                                n180 = Negate(x=w198) -> (-x=w193:dbl)
                                n181 = Select(t=0.0, s=w196, f=w193) -> (s? t:f=→"lane_shift":dbl)
                              }
                            }
                          }
                          frame #1 {
                            w225 = 0.98 ("Shift LPF gain")
                            n182 = feedback-in #4("lane keep") -> ()
                            n183 = feedback #4("lane keep") -> (w234:bool)
                            n184 = Not Equal?(x="lane keep", y=w234) -> (x != y?=w233:bool)
                            n185 = And(x="lane keep", y=w233) -> (x .and. y?=w231:bool)
                            n186 = case shown="False" w231 {
                              tunnel: [w242 _] -> w230
                              frame False {
                                n187 = local read "x"() -> (w242:dbl)
                              }
                              frame True {
                                n188 = local write "x"(0.0 ("x")) -> ()
                              }
                            }
                            n189 = local read "lane_shift"() -> (w221:dbl)
                            n190 = local read "x"() -> (w223:dbl)
                            n191 = Multiply(x=w223, y=0.5) -> (x*y=w222:dbl)
                            n192 = Add(x=w221, y=w222) -> (x+y=w220:dbl)
                            n193 = feedback #5(w220) -> (w226:dbl)
                            n194 = Decrement(x=w225) -> (x-1=w227:dbl)
                            n195 = Multiply(x=w230, y=0.5) -> (x*y=w239:dbl)
                            n196 = local read "obs shift"() -> (w236:dbl)
                            n197 = Multiply(x=w226, y=w225) -> (x*y=w228:dbl)
                            n198 = Multiply(x=w227, y=w220) -> (x*y=w229:dbl)
                            n199 = Select(t=w239, s="lane keep", f=0.0) -> (s? t:f=w237:dbl)
                            n200 = Add(x=w236, y=w237) -> (x+y=w235:dbl)
                            n201 = Subtract(x=w228, y=w229) -> (x-y=w241:dbl)
                            n202 = feedback-in #5(w241) -> ()
                            n203 = call "tracking1.vi"("lane keep"="lane keep", "xbody"=w235, "xt"=w241) -> ("handle"=w217:dbl)  [unwired: 7 in, 1 out]
                            n204 = Multiply(x=w217, y="Steering gain") -> (x*y=w219:dbl)
                            n205 = global write "G_VEH.vi" "handle"(w219) -> ()
                          }
                          frame #2 {
                            n206 = global read "G_SEN.vi" "sensor_obs"() -> (w258:dbl[][])
                            n207 = global read "G_PATH.vi" "map_track"() -> (w257:dbl[][])
                            n208 = for {
                              tunnel: w257 -> [w304] mode=indexing
                              tunnel: w258 -> [w306]
                              tunnel: [w291] -> w264 mode=indexing
                              tunnel: [w293] -> w265 mode=indexing
                              stop <- w290 stop-if-true
                              n209 = Index Array(array=w304, index #1=0 ("index")) -> (element #1=w302:dbl, element #2=w300:dbl)  [unwired: 1 in]
                              n210 = Index Array(array=w306, index (col) #1=0 ("disabled index (col)")) -> (element #1=w301:dbl[], element #2=w299:dbl[])  [unwired: 3 in]
                              n211 = Subtract(x=w302, y=w301) -> (x-y=w298:dbl[])
                              n212 = Subtract(x=w300, y=w299) -> (x-y=w297:dbl[])
                              n213 = Square(x=w298) -> (x^2=w296:dbl[])
                              n214 = Square(x=w297) -> (x^2=w295:dbl[])
                              n215 = Add(x=w296, y=w295) -> (x+y=w294:dbl[])
                              n216 = local read "half width"() -> (w292:dbl)
                              n217 = Array Max & Min(array=w294) -> (min value=w291:dbl, min index (indices)=w293:i32)  [unwired: 2 out]
                              n218 = Greater?(x=w292, y=w291) -> (0:w290:bool)
                            }
                            n219 = Array Max & Min(array=w264) -> (min value=w251:dbl, min index (indices)=w256:i32)  [unwired: 2 out]
                            n220 = Square Root(x=w251) -> (sqrt(x)=w247:dbl)
                            n221 = Index Array(array=w257, index (row)=w256) -> (element=w255:dbl[])  [unwired: 1 in]
                            n222 = Index Array(array=w265, index=w256) -> (element=w261:i32)
                            n223 = Index Array(array=w258, index (row)=w261) -> (element=w253:dbl[])  [unwired: 1 in]
                            n224 = Subtract(x=w255, y=w253) -> (x-y=w252:dbl[])
                            n225 = Index Array(array=w253, index #1=0 ("index")) -> (element #1=w254:dbl, element #2=w259:dbl)  [unwired: 1 in]
                            n226 = In Range and Coerce(upper limit="half width", x=w247, lower limit=0.5) -> (In Range?=w249:bool)  [unwired: 1 out]
                            n227 = global read "G_VEH.vi" "xtmp"() -> (w262:T5)
                            n228 = Index Array(array=w252) -> (element=w248:dbl)  [unwired: 1 in]
                            n229 = Bundle By Name(cluster=w262, "x"=w254, "y"=w259) -> (w263:T5)
                            n230 = case shown="False" w249 {
                              tunnel: w248 -> [_ w289]
                              tunnel: [w281 w286] -> w246
                              tunnel: w247 -> [w283 _]
                              tunnel: "shifthold" -> [w266 w285]
                              frame False {
                                n231 = Negate(x=w266) -> (-x=w267:dbl)
                                n232 = local read "half width"() -> (w271:dbl)
                                n233 = local read "obs shift"() -> (w278:dbl)
                                n234 = Sign(1:w278) -> (0:w280:dbl)
                                n235 = Multiply(x=w271, y=0.1) -> (x*y=w269:dbl)
                                n236 = Multiply(x=w280, y=w267) -> (x*y=w279:dbl)
                                n237 = Add(x=w271, y=w269) -> (x+y=w268:dbl)
                                n238 = Add(x=w278, y=w279) -> (x+y=w274:dbl)
                                n239 = Greater?(x=w283, y=w268) -> (0:w282:bool)
                                n240 = Absolute Value(x=w274) -> (abs(x)=w277:dbl)
                                n241 = Greater?(x=w277, y=0.01) -> (0:w275:bool)
                                n242 = Select(t=w274, s=w275, f=0.0) -> (s? t:f=w272:dbl)
                                n243 = Select(t=w272, s=w282, f=w278) -> (s? t:f=w281:dbl)
                              }
                              frame True {
                                n244 = Sign(1:w289) -> (0:w284:dbl)
                                n245 = local read "obs shift"() -> (w287:dbl)
                                n246 = Multiply(x=w285, y=w284) -> (x*y=w288:dbl)
                                n247 = Add(x=w287, y=w288) -> (x+y=w286:dbl)
                              }
                            }
                            "obs shift" <- w246
                            n248 = global write "G_VEH.vi" "xtmp"(w263) -> ()
                          }
                        }
                      }
                      frame Disabled {
                      }
                    }
                  }
                  frame True {
                    n249 = flat-sequence {
                      frame #0 {
                        w308 = FALSE ("X Scale.Loose Fit")
                        w307 = u8 0 ("X Scale.Scale Fit")
                        n250 = call "initvar.vi"() -> ()  [unwired: 12 in]
                        n251 = property on="XY Graph" class="XYGraph (strict)"("XScale.ScaleFit"=w307, "YScale.ScaleFit"=w307, "XScale.LooseFit"=w308, "YScale.LooseFit"=w308) -> ()  [unwired: 2 in, 2 out]
                      }
                      frame #1 {
                        n252 = global read "G_VEH.vi" "Location"() -> (w309:i32)
                        n253 = Bundle("Minimum"=-5.0, "Minimum"=37.3, "Minimum"=10.0, "Minimum"=1.0, "Minimum"=-20.0) -> (w315:T12)  [unwired: 1 in]
                        n254 = Bundle("Minimum"=-22.6, "Minimum"=22.6, "Minimum"=10.0, "Minimum"=1.0, "Minimum"=-20.0) -> (w322:T12)  [unwired: 1 in]
                        n255 = call "getecefdcmref.vi"("map"=w309) -> ("XYZ"=w310:dbl[])  [unwired: 10 in, 4 out]
                        n256 = property on="XY Graph" class="XYGraph (strict)"("XScale.Range"=w322) -> ()  [unwired: 2 in, 2 out]
                        n257 = property on="XY Graph" class="XYGraph (strict)"("YScale.Range"=w315) -> ()  [unwired: 2 in, 2 out]
                        n258 = global write "G_NAV.vi" "ecef ref"(w310) -> ()
                      }
                      frame #2 {
                        n259 = global read "G_DATA.vi" "path"() -> (w326:path)
                        n260 = Build Path(base path=w326, name or relative path="wpt") -> (appended path=w324:path)
                        n261 = call "Read From Measurement File2"("Filename"=w324, "Reset"=TRUE) -> ("error out"=w328:errorcluster, "Filename Out"=w323:path, "Signals"=w330:dynamicdata)  [unwired: 4 in, 3 out]
                        n262 = Unbundle By Name(w328) -> ("status"=w327:bool)
                        n263 = case shown="False" w327 {
                          tunnel: w330 -> [w332 _]
                          tunnel: w323 -> [w331 _]
                          frame False {
                            n264 = call "Convert from Dynamic Data2"("Dynamic Data Type"=w332) -> ("Array"=w334:dbl[][])  [unwired: 3 in]
                            n265 = Empty Array?(array=w334) -> (empty?=w333:bool)
                            n266 = case shown="False" w333 {
                              tunnel: w334 -> [w336 _]
                              tunnel: w331 -> [w335 _]
                              frame False {
                                n267 = call "path_ini_new.vi"("Filename Out"=w335, "WPT"=w336) -> ()  [unwired: 10 in]
                              }
                              frame True {
                                w337 = dbl[][] [] ("path_updated")
                                n268 = global write "G_PATH.vi" "path"(w337) -> ()
                                n269 = global write "G_PATH.vi" "path_very_origin"(w337) -> ()
                                n270 = global write "G_PATH.vi" "path_origin"(w337) -> ()
                              }
                            }
                          }
                          frame True {
                            w338 = dbl[][] [] ("path_updated")
                            n271 = global write "G_PATH.vi" "path"(w338) -> ()
                            n272 = global write "G_PATH.vi" "path_very_origin"(w338) -> ()
                            n273 = global write "G_PATH.vi" "path_origin"(w338) -> ()
                          }
                        }
                      }
                      frame #3 {
                        w339 = T13 [] ("Missions_origin")
                        n274 = global read "G_VEH.vi" "Location"() -> (w340:i32)
                        n275 = local write "Load WPT"(FALSE ("Load WPT")) -> ()
                        n276 = global write "G_PATH.vi" "Missions_origin"(w339) -> ()
                        n277 = global write "G_PATH.vi" "Missions"(w339) -> ()
                        n278 = call "mapconf.vi"("Location"=w340) -> ("y"=w342:cluster{dbl, dbl, "y":dbl, "y":dbl, dbl}, "x"=w343:cluster{dbl, dbl, "y":dbl, "y":dbl, dbl}, "new picture"=w344:picture)  [unwired: 8 in]
                        n279 = property on="XY Graph 2" class="XYGraph (strict)"("PlotImages.Back"=w344) -> ()  [unwired: 2 in, 2 out]
                        n280 = property on="XY Graph 2" class="XYGraph (strict)"("XScale.Range"=w343, "YScale.Range"=w342) -> ()  [unwired: 2 in, 2 out]
                      }
                    }
                  }
                }
              }
              frame True {
                n281 = flat-sequence {
                  tunnel: [w349] -> w345
                  tunnel: w345 -> [w438]
                  frame #0 {
                    w346 = 0.0
                    n282 = global write "G_VEH.vi" "handle"(w346) -> ()
                    n283 = global write "G_VEH.vi" "VS_des"(w346) -> ()
                  }
                  frame #1 {
                    n284 = local read "Make WPT"() -> (w348:bool)
                    n285 = global read "G_VEH.vi" "Location"() -> (w347:i32)
                    n286 = Initialize Array(0.0 ("element"), 7 ("dimension size"), 1 ("dimension size")) -> (w350:dbl[][])
                    n287 = while {
                      shift-right: [w355] -> w349
                      shift-left: w350 -> [w357]
                      shift-right: [FALSE] -> _
                      shift-left: w348 -> [w358]
                      tunnel: w347 -> [w354]
                      stop <- w360 stop-if-true
                      n288 = flat-sequence {
                        tunnel: [w370] -> w356
                        tunnel: w354 -> [w363]
                        frame #0 {
                          n289 = global read "G_NAV.vi" "GPS_status"() -> (w362:T14)
                          n290 = disable-structure shown="Enabled" {
                            disable-tunnel: [w381 w385] -> w373
                            disable-tunnel: [w380 w384] -> w372
                            disable-tunnel: [w374 w383] -> w371
                            disable-tunnel: w362 -> [w379 w393]
                            disable-tunnel: [w378 w392] -> w369
                            disable-tunnel: [w377 w391] -> w368
                            disable-tunnel: [w374 w390] -> w367
                            disable-tunnel: w363 -> [_ w389]
                            frame Enabled {
                              n291 = Unbundle By Name(w379) -> ("lat"=w378:dbl, "lon"=w377:dbl, "hgt"=w374:dbl)
                              n292 = global read "G_NAV.vi" "M6006"() -> (w382:T11)
                              n293 = Unbundle By Name(w382) -> ("lcc[0]"=w376:dbl, "lcc[1]"=w375:dbl)
                              n294 = To Double Precision Float(number=w376) -> (double precision float=w381:dbl)
                              n295 = To Double Precision Float(number=w375) -> (double precision float=w380:dbl)
                            }
                            frame Disabled {
                              n296 = Unbundle By Name(w393) -> ("lat"=w392:dbl, "lon"=w391:dbl, "hgt"=w390:dbl)
                              n297 = call "getecefdcmref.vi"("map"=w389) -> ("XYZ"=w388:dbl[])  [unwired: 10 in, 4 out]
                              n298 = call "llh2lcc.vi"("ecef ref"=w388, "hgt"=w390, "lon"=w391, "lat"=w392) -> ("lcc"=w387:dbl[])  [unwired: 7 in]
                              n299 = Index Array(array=w387, index #1=0 ("index")) -> (element #1=w385:dbl, element #2=w384:dbl, element #3=w383:dbl)  [unwired: 2 in]
                            }
                          }
                          n300 = To Double Precision Float(number=w363) -> (double precision float=w364:dbl)
                          n301 = global read "G_VEH.vi" "candata"() -> (w366:T10)
                          n302 = Unbundle By Name(w366) -> ("VS_can"=w365:dbl)
                          n303 = Build Array(w369, w368, w367, w373, w372, w371, w365, w364) -> (w370:dbl[])
                        }
                      }
                      n304 = local read "Make WPT"() -> (w361:bool)
                      n305 = Not(x=w361) -> (.not. x?=w360:bool)
                      n306 = case shown="False" w358 {
                        tunnel: w357 -> [w408 w425]
                        tunnel: w356 -> [w407 w423]
                        tunnel: [w406 w422] -> w355
                        frame False {
                          n307 = Array Size(array=w408) -> (size(s)=w416:i32[])
                          n308 = Index Array(array=w407, index #1=3 ("index"), index #2=4 ("index")) -> (element #1=w402:dbl, element #2=w400:dbl)
                          n309 = Index Array(array=w416, index=1) -> (element=w405:i32)
                          n310 = Decrement(x=w405) -> (x-1=w404:i32)
                          n311 = Index Array(array=w408, index (col)=w404) -> (element=w412:dbl[])  [unwired: 1 in]
                          n312 = Index Array(array=w412, index #1=3 ("index"), index #2=4 ("index")) -> (element #1=w403:dbl, element #2=w401:dbl)
                          n313 = Subtract(x=w403, y=w402) -> (x-y=w399:dbl)
                          n314 = Subtract(x=w401, y=w400) -> (x-y=w398:dbl)
                          n315 = Square(x=w399) -> (x^2=w397:dbl)
                          n316 = Square(x=w398) -> (x^2=w396:dbl)
                          n317 = Add(x=w397, y=w396) -> (x+y=w395:dbl)
                          n318 = Greater Or Equal?(x=w395, y=0.25) -> (x >= y?=w409:bool)
                          n319 = case shown="True" w409 {
                            tunnel: w408 -> [w417 w421]
                            tunnel: w405 -> [_ w418]
                            tunnel: w407 -> [_ w420]
                            tunnel: [w417 w419] -> w406
                            frame False {
                            }
                            frame True {
                              n320 = Insert Into Array(array=w421, index (col)=w418, new element=w420) -> (w419:dbl[][])  [unwired: 1 in]
                            }
                          }
                        }
                        frame True {
                          n321 = Replace Array Subset(array=w425, new element=w423, index (col)=0 ("disabled index (col)")) -> (w422:dbl[][])  [unwired: 1 in]
                        }
                      }
                    }
                  }
                  frame #2 {
                    n322 = call "Convert to Dynamic Data"("2D Array"=w438) -> ("Dynamic Data Type"=w439:dynamicdata)  [unwired: 3 in]
                    n323 = global read "G_VEH.vi" "Location"() -> (w435:i32)
                    n324 = case shown="9" w435 {
                      tunnel: ["" ("String") "Hyundai" ("String") "KAIST" ("String") "AJOU" ("String") "MUNJI" ("String") "Airforce" ("String") "CAR" ("String") "KATRI" ("String") _ "coex" ("String")] -> w434
                      frame 0, Default {
                      }
                      frame 1 {
                      }
                      frame 2 {
                      }
                      frame 3 {
                      }
                      frame 4 {
                      }
                      frame 5 {
                      }
                      frame 6 {
                      }
                      frame 7 {
                      }
                      frame 8 {
                      }
                      frame 9 {
                      }
                    }
                    n325 = Get Date/Time In Seconds() -> (seconds since 1Jan1904=w436:timestamp)
                    n326 = Format Date/Time String(time format string (%c)="%2y%2m%2d%2H%2M", seconds (now)=w436) -> (date/time string=w432:string)  [unwired: 1 in]
                    n327 = global read "G_DATA.vi" "path"() -> (w430:path)
                    n328 = Build Path(base path=w430, name or relative path="wpt") -> (appended path=w428:path)
                    n329 = Concatenate Strings(w432, "_" ("string"), w434, ".lvm" ("string")) -> (w427:string)
                    n330 = Build Path(base path=w428, name or relative path=w427) -> (appended path=w426:path)
                    n331 = call "save wpt"("Signals"=w439, "Reset"=TRUE, "Filename"=w426) -> ()  [unwired: 14 in, 3 out]
                  }
                }
              }
            }
          }
        }
      }
    }
  }
  n332 = flat-sequence {
    frame #0 {
      # "Sensor paser"
    }
    frame #1 {
      w451 = dbl[][] [] ("sensor_car")
      w452 = dbl[][] [] ("sensor_lane_log")
      n333 = disable-structure shown="Enabled" {
        disable-tunnel: [dbl[][] array18932x2[37864 elements] ("all rows") _] -> w450
        frame Disabled {
        }
        frame Enabled {
        }
      }
      n334 = local write "Log"(FALSE ("obs")) -> ()
      n335 = global write "G_SEN.vi" "data"(w451) -> ()
      n336 = global write "G_SEN.vi" "sensor_lane_log"(w452) -> ()
      n337 = global write "G_SEN.vi" "sensor_obs_log"(w452) -> ()
      n338 = global write "G_SEN.vi" "sensor_etc"(w451) -> ()
      n339 = global write "G_SEN.vi" "sensor_lane"(w451) -> ()
      n340 = global write "G_SEN.vi" "sensor_obs"(w451) -> ()
      n341 = global write "G_SEN.vi" "map_lane"(w450) -> ()
    }
    frame #2 {
      n342 = while {
        stop <- FALSE stop-if-true
        n343 = flat-sequence {
          frame #0 {
            n344 = Wait Until Next ms Multiple(millisecond multiple=u32 10 ("milliseconds to wait")) -> (millisecond timer value=w456:u32)
            n345 = feedback #6() -> (w458:u32)  [unwired: 1 in]
            n346 = feedback-in #6(w456) -> ()
            n347 = Subtract(x=w456, y=w458) -> (x-y=→"sensor":u32)
          }
          frame #1 {
            n348 = disable-structure shown="Enabled" {
              frame Enabled {
                w460 = 0.0 ("roll")
                n349 = call "velodynepaser.vi"("roll"=w460, "pitch"=w460, "heading"=w460, "dX"=w460, "dY"=w460, "dZ"=w460) -> ()  [unwired: 12 in, 2 out]
              }
              frame Disabled {
              }
            }
            n350 = disable-structure shown="Enabled" {
              frame Enabled {
                n351 = call "mobileyelanepaser4.vi"("count hold"=u64 15, "thresh  c"=0.5, "thresh  b"=0.06 ("thresh 2"), "thresh r"=0.009 ("y")) -> ()  [unwired: 4 in, 4 out]
                n352 = call "mobileyepaser.vi"() -> ()  [unwired: 11 in, 1 out]
              }
              frame Disabled {
              }
            }
          }
          frame #2 {
            w467 = TRUE ("Sensor [F12]")
            n353 = global read "G_SEN.vi" "M_lane_update"() -> (→"update":bool)
            n354 = call "Ibeopaser.vi"("theta"=-2.5, "Hide Transparent"=w467, "Sensor [F12]"=w467) -> ("x_sensor"=w471:T5, "etc"=w469:dbl[][], "lane"=w470:dbl[][], "obs"=w472:dbl[][], "update"=w468:bool)  [unwired: 4 in]
            n355 = case shown="True" w468 {
              tunnel: w472 -> [_ w477]
              tunnel: w471 -> [_ w478]
              tunnel: w470 -> [_ w474]
              tunnel: w469 -> [_ w475]
              frame False {
              }
              frame True {
                n356 = disable-structure shown="Enabled" {
                  disable-tunnel: w477 -> [w483 w485]
                  disable-tunnel: [w482 w485] -> w476
                  disable-tunnel: w475 -> [w481 _]
                  disable-tunnel: w474 -> [w480 w484]
                  disable-tunnel: [w479 w484] -> w473
                  frame Disabled {
                    n357 = call "test3.vi"("sensor_all"=w481, "sensor_lane"=w480, "sensor_obs"=w483) -> ("lane"=w479:dbl[][], "obs"=w482:dbl[][])  [unwired: 6 in, 1 out]
                  }
                  frame Enabled {
                  }
                }
                n358 = global write "G_VEH.vi" "xsensor"(w478) -> ()
                n359 = global write "G_SEN.vi" "sensor_obs"(w476) -> ()
                n360 = global write "G_SEN.vi" "sensor_lane"(w473) -> ()
              }
            }
          }
          frame #3 {
            n361 = case shown="True" "Log" {
              frame False {
                n362 = global write "G_SEN.vi" "sensor_obs_log"(dbl[][] [] ("sensor_obs_log")) -> ()
              }
              frame True {
                n363 = global read "G_VEH.vi" "candata"() -> (w489:T10)
                n364 = Unbundle By Name(w489) -> ("VS_can"=w490:dbl)
                n365 = Not Equal To 0?(x=w490) -> (x != 0?=w488:bool)
                n366 = case shown="True" w488 {
                  frame False {
                  }
                  frame True {
                    n367 = global read "G_SEN.vi" "sensor_obs_log"() -> (w492:dbl[][])
                    n368 = global read "G_SEN.vi" "sensor_obs"() -> (w493:dbl[][])
                    n369 = call "sensor_log2.vi"("xmax"=8.0, "range^2"=16.0, "xmin"=-5.0, "FF"=0.93 ("t"), "ymin"=0.0, "ymax"=20.0, "sensor_log"=w492, "sensor_obs"=w493) -> ("sensor_log 2"=w491:dbl[][])  [unwired: 2 in, 1 out]
                    n370 = global write "G_SEN.vi" "sensor_obs_log"(w491) -> ()
                  }
                }
              }
            }
          }
          frame #4 {
            n371 = disable-structure shown="Enabled" {
              frame Enabled {
                n372 = global read "G_VEH.vi" "candata"() -> (w506:T10)
                n373 = global read "G_VEH.vi" "sys time"() -> (w501:i64)
                n374 = Unbundle By Name(w506) -> ("VS_can"=w507:dbl)
                n375 = feedback-in #7(w501) -> ()
                n376 = feedback #7(i64 0 ("sys time")) -> (w505:i64)
                n377 = Not Equal To 0?(x=w507) -> (x != 0?=w503:bool)
                n378 = Greater?(x=w501, y=w505) -> (0:w504:bool)
                n379 = And(x=w503, y=w504) -> (x .and. y?=w502:bool)
                n380 = case shown="True" w502 {
                  frame False {
                  }
                  frame True {
                    n381 = flat-sequence {
                      tunnel: [w509] -> w508
                      tunnel: w508 -> [w527]
                      frame #0 {
                        n382 = disable-structure shown="Enabled" {
                          disable-tunnel: [50.0 ("ymax") 10000.0 ("ymax")] -> w514
                          disable-tunnel: [-3.5 ("ymin") -10000.0 ("ymin")] -> w513
                          disable-tunnel: [-6.0 ("xmin") -10000.0 ("xmin")] -> w512
                          disable-tunnel: [10.0 ("xmin") 10000.0 ("xmax")] -> w511
                          frame Enabled {
                          }
                          frame Disabled {
                          }
                        }
                        n383 = global read "G_SEN.vi" "sensor_lane_log"() -> (w518:dbl[][])
                        n384 = global read "G_SEN.vi" "sensor_lane"() -> (w517:dbl[][])
                        n385 = call "sensor_log2.vi"("xmax"=w511, "range^2"=0.0, "xmin"=w512, "FF"=1.0, "ymin"=w513, "ymax"=w514, "sensor_log"=w518, "sensor_obs"=w517) -> ("sensor_log_body"=w509:dbl[][], "sensor_log 2"=w510:dbl[][])  [unwired: 2 in]
                        n386 = global write "G_SEN.vi" "sensor_lane_log"(w510) -> ()
                      }
                      frame #1 {
                        n387 = disable-structure shown="Enabled" {
                          disable-tunnel: w527 -> [w528 _]
                          frame Disabled {
                            n388 = call "lane_test1.vi"("lane_body"=w528) -> ()  [unwired: 11 in]
                          }
                          frame Enabled {
                          }
                        }
                      }
                    }
                  }
                }
              }
              frame Disabled {
              }
            }
          }
        }
      }
    }
  }
